vi "Case.vi"() -> ()   [LabVIEW 2018]
panel:
  in  "문자열":string="키다"
  in  "숫자형":i32
  in  "불리언":bool=TRUE
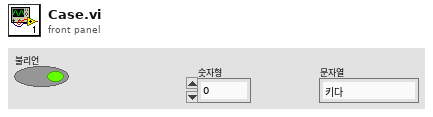
[diagram p1: front panel]
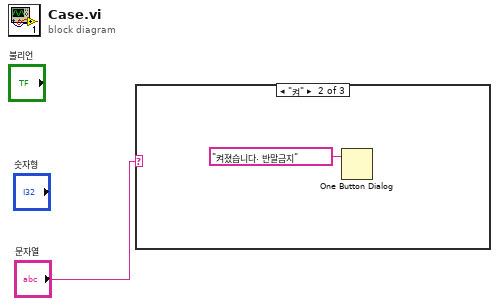
[diagram p0: block diagram]
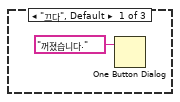
[diagram p2: hidden frame]
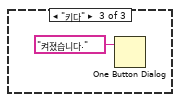
[diagram p3: hidden frame]
diagram:
  n1 = case shown="\"켜\"" "문자열" {
    frame "끄다", Default {
      n2 = One Button Dialog(message="꺼졌습니다." ("메시지")) -> ()  [unwired: 1 in, 1 out]
    }
    frame "켜" {
      n3 = One Button Dialog(message="켜졌습니다. 반말금지" ("메시지")) -> ()  [unwired: 1 in, 1 out]
    }
    frame "키다" {
      n4 = One Button Dialog(message="켜졌습니다." ("메시지")) -> ()  [unwired: 1 in, 1 out]
    }
  }
